vi "MeasureLeq.vi"(0 "channel info left(necessary)":T4={"sensor sensitivity"=12.21, "engineering units"=2, "dB reference"=2e-05, "pregain"=0.0} {"pregain" format="%.2f"; "dB reference" format="%^.1e"; "engineering units" items=["custom..."=0, "V"=1, "A"=21, "C"=30, "pC"=31, "s"=32, "-"=29, "Pa"=2, "N"=20, "g"=3, "m/s^2"=4, "m/s"=5, "m"=6, "mm/s"=12, "mm"=13, "micron/s"=14, "micron"=15, "in/s^2"=7, "in/s"=8, "in"=9, "mil/s"=10, "mil"=11, "rad/s^2"=16, "rad/s"=17, "rad"=18, "deg/s^2"=26, "deg/s"=27, "deg"=28, "RPM"=22, "cycle/s^2"=23, "Hz"=24, "cycle"=25, "strain"=19]; "sensor sensitivity" format="%#_5f"}, 1 "channel info right (necessary)":T4={"sensor sensitivity"=13.0, "engineering units"=2, "dB reference"=2e-05, "pregain"=0.0} caption="channel info right(necessary)" {"pregain" format="%.2f"; "dB reference" format="%^.1e"; "engineering units" items=["custom..."=0, "V"=1, "A"=21, "C"=30, "pC"=31, "s"=32, "-"=29, "Pa"=2, "N"=20, "g"=3, "m/s^2"=4, "m/s"=5, "m"=6, "mm/s"=12, "mm"=13, "micron/s"=14, "micron"=15, "in/s^2"=7, "in/s"=8, "in"=9, "mil/s"=10, "mil"=11, "rad/s^2"=16, "rad/s"=17, "rad"=18, "deg/s^2"=26, "deg/s"=27, "deg"=28, "RPM"=22, "cycle/s^2"=23, "Hz"=24, "cycle"=25, "strain"=19]; "sensor sensitivity" format="%#_5f"}, 3 "sample mode":T9 items=["Finite Samples", "Continuous Samples"], 8 "path":path=path "C:/Users/eeeds/OneDrive/Desktop/white noise30s.wav", 9 "device ID":u32, 10 "task":refnum<k21>, 12 "Amplification":dbl=1.0, 14 "weighting 2":u16(ring)=1 items=["Linear", "A-weighting", "B-weighting", "C-weighting"], 16 "weighting 3":u16(ring)=1 items=["Linear", "A-weighting", "B-weighting", "C-weighting"]) -> (20 "Leq sound level [dB EU] 4":dbl format="%.1f", 22 "max value":dbl, 24 "iterations":i32 caption="Numeric")   [LabVIEW 2019]
uses:
  <vilib>/addons/_NISVFA/_Shared subVIs/Controls/svc_Engineering Units Text Ring.ctl
  <vilib>/addons/_NISVFA/_Shared subVIs/Controls/svc_Window.ctl
  <vilib>/sound2/lvsound2.llb/Sampling Mode.ctl
  <vilib>/addons/_NISVFA/_Shared subVIs/Controls/svc_Weighting Filter Text Ring.ctl
  <vilib>/Utility/error.llb/DialogType.ctl
  <vilib>/DAQmx/read.llb/DAQmx Read (Analog 1D Wfm NChan NSamp).vi
  <vilib>/addons/Sound and Vibration/svt_Calibration/SVL Scale Voltage to EU (N Ch - N Info).vi
  <vilib>/addons/Sound and Vibration/svt_Calibration/SVL Scale Voltage to EU (1 Ch).vi
  <vilib>/addons/_NISVFA/_Shared subVIs/Common/svc_Set SV Channel Info.vi
  <vilib>/addons/_NISVFA/_Shared subVIs/Common/svc_Set SV Channel Info (variant).vi
  <vilib>/addons/_NISVFA/_Shared subVIs/Common/SVL Set dB Reference (variant).vi
  <vilib>/sound2/lvsound2.llb/Sound File Info (path).vi
  GlobalVariable.vi
  <vilib>/DAQmx/miscellaneous.llb/DAQmx Fill In Error Info.vi
  <vilib>/addons/_NISVFA/_Shared subVIs/Common/svc_Engineering Units to Unit Label.vi
  <vilib>/addons/_NISVFA/_Shared subVIs/Common/svc_Compute Scale Factor to Convert V to EU.vi
  <vilib>/addons/_NISVFA/_Shared subVIs/Common/svc_Compute Scale Factor to Convert C to EU.vi
  <vilib>/addons/_NISVFA/_Shared subVIs/Common/svc_Set dB ref if Pascal.vi
  <vilib>/addons/_NISVFA/_Shared subVIs/Common/svc_Caller VI Returned in Error Source.vi
  <vilib>/Waveform/WDTOps.llb/WDT Index Channel DBL.vi
  <vilib>/addons/Sound and Vibration/svt_Weighting/SVT Weighting Filter (1 Ch).vi
  <vilib>/addons/Sound and Vibration/svt_Octave_2014 standard/SVT Third-octave Analysis (1 Ch).vi
  <vilib>/addons/Sound and Vibration/svt_Level/SVL RMS Level (N Ch).vi
  <vilib>/addons/Sound and Vibration/svt_Octave/SVT Third-octave Analysis (N Ch).vi
  <vilib>/addons/_NISVFA/_Baseband FFT/SVFA Power Spectrum (N Ch).vi
  <vilib>/addons/_NISVFA/_Zoom FFT/SVFA Zoom Power Spectrum (N Ch).vi
  <vilib>/addons/_NISVFA/_Subset FFT/SVFA Power Spectrum Subset (N Ch).vi
  <vilib>/addons/_NISVFA/_Baseband FFT/SVFA FFT Spectrum (Mag-Phase) (N Ch).vi
  <vilib>/addons/_NISVFA/_Zoom FFT/SVFA Zoom FFT Spectrum (Mag-Phase) (N Ch).vi
  <vilib>/addons/_NISVFA/_Subset FFT/SVFA FFT Spectrum Subset (Mag-Phase) (N Ch).vi
  <vilib>/addons/_NISVFA/_Baseband FFT/SVFA Power Spectral Density (N Ch).vi
  <vilib>/addons/_NISVFA/_Zoom FFT/SVFA Zoom Power Spectral Density (N Ch).vi
  <vilib>/addons/_NISVFA/_Subset FFT/SVFA Power Spectral Density Subset (N Ch).vi
  <vilib>/addons/Sound and Vibration/svt_Level/SVT Sound Level (1 Ch).vi
  <vilib>/sound2/lvsound2.llb/Sound Output Write (DBL).vi
  <vilib>/addons/Sound and Vibration/svt_Calibration/SoundVib_Calibration.lvlib
  <vilib>/addons/Sound and Vibration/svt_Octave/SoundVib_Octave.lvlib
  <vilib>/addons/Sound and Vibration/svt_Level/SoundVib_VibrationLevel.lvlib
  <vilib>/addons/Sound and Vibration/svt_Weighting/SoundVib_ABCWeighting.lvlib
  <vilib>/addons/Sound and Vibration/svt_Level/SoundVib_SoundLevel.lvlib
  <vilib>/addons/Sound and Vibration/svt_Octave/SoundVib_Octave_2014 standard.lvlib
  <resource>/objmgr/daqmx.rc
panel:
  out "time*10":i16
  in  "channel info right 2(unnecessary)":T2={"weighting filter 2"=0, "custom label"="EU"} {"weighting filter 2" items=["Linear", "A-weighting", "B-weighting", "C-weighting", "ITU-R 468-4", "Dolby", "CCITT", "C-message", "Wb", "Wc", "Wd", "We", "Wf", "Wh", "Wj", "Wk", "Wm", "AES17 20 kHz lowpass", "AES17 40 kHz lowpass", "AES17 20 kHz highpass", "AES17 40 kHz highpass"]}
  in  "channel info left":T5={"sensor sensitivity"=12.21, "engineering units"=2, "dB reference"=2e-05, "custom label"="EU", "weighting filter"=0, "pregain"=0.0} {"pregain" format="%.2f"; "weighting filter" items=["Linear", "A-weighting", "B-weighting", "C-weighting", "ITU-R 468-4", "Dolby", "CCITT", "C-message", "Wb", "Wc", "Wd", "We", "Wf", "Wh", "Wj", "Wk", "Wm", "AES17 20 kHz lowpass", "AES17 40 kHz lowpass", "AES17 20 kHz highpass", "AES17 40 kHz highpass"]; "dB reference" format="%^.1e"; "engineering units" items=["custom..."=0, "V"=1, "A"=21, "C"=30, "pC"=31, "s"=32, "-"=29, "Pa"=2, "N"=20, "g"=3, "m/s^2"=4, "m/s"=5, "m"=6, "mm/s"=12, "mm"=13, "micron/s"=14, "micron"=15, "in/s^2"=7, "in/s"=8, "in"=9, "mil/s"=10, "mil"=11, "rad/s^2"=16, "rad/s"=17, "rad"=18, "deg/s^2"=26, "deg/s"=27, "deg"=28, "RPM"=22, "cycle/s^2"=23, "Hz"=24, "cycle"=25, "strain"=19]; "sensor sensitivity" format="%#_5f"}
  in  "channel info left (unnecessary)":T2={"weighting filter 2"=0, "custom label"="EU"} {"weighting filter 2" items=["Linear", "A-weighting", "B-weighting", "C-weighting", "ITU-R 468-4", "Dolby", "CCITT", "C-message", "Wb", "Wc", "Wd", "We", "Wf", "Wh", "Wj", "Wk", "Wm", "AES17 20 kHz lowpass", "AES17 40 kHz lowpass", "AES17 20 kHz highpass", "AES17 40 kHz highpass"]}
  out "number of channels":dbl
  out "bits per sample":dbl
  out "sample rate":dbl
  in  "channel info right":T5={"sensor sensitivity"=13.0, "engineering units"=2, "dB reference"=2e-05, "custom label"="EU", "weighting filter"=0, "pregain"=0.0} {"pregain" format="%.2f"; "weighting filter" items=["Linear", "A-weighting", "B-weighting", "C-weighting", "ITU-R 468-4", "Dolby", "CCITT", "C-message", "Wb", "Wc", "Wd", "We", "Wf", "Wh", "Wj", "Wk", "Wm", "AES17 20 kHz lowpass", "AES17 40 kHz lowpass", "AES17 20 kHz highpass", "AES17 40 kHz highpass"]; "dB reference" format="%^.1e"; "engineering units" items=["custom..."=0, "V"=1, "A"=21, "C"=30, "pC"=31, "s"=32, "-"=29, "Pa"=2, "N"=20, "g"=3, "m/s^2"=4, "m/s"=5, "m"=6, "mm/s"=12, "mm"=13, "micron/s"=14, "micron"=15, "in/s^2"=7, "in/s"=8, "in"=9, "mil/s"=10, "mil"=11, "rad/s^2"=16, "rad/s"=17, "rad"=18, "deg/s^2"=26, "deg/s"=27, "deg"=28, "RPM"=22, "cycle/s^2"=23, "Hz"=24, "cycle"=25, "strain"=19]; "sensor sensitivity" format="%#_5f"}
  in  "quit 4":bool
  in  "exp avg settings 4":T6={" mode"=enum."Fast", "time constant [ms]"=125.0} {"time constant [ms]" format="%.2f"}
  in  "frequency range 4":T7={"low band"=enum."20 Hz", "high band"=enum."16000 Hz"}
  out "filter settled 3":bool
  out "octave graph 3":T8(graph)
  out "Total Band Power 3":dbl(slide)=nan scale=0.0..100.0
  out "History 3":waveform(dbl)[](graph)
  out "Leq sound level [dB EU] 3":dbl format="%.1f"
  out "unit label 3":string="left dB(A) ref 20.0u Pa" caption="Left"
  out "Exp Avg 3":dbl format="%.1f"
  in  "restart 4":bool
  in  "integration time [s] 2":dbl=10.0 format="%.2f"
  out "Running Leq sound level [dB EU] 4":dbl format="%.1f"
  out "Running Leq sound level [dB EU] 3":dbl format="%.1f"
  in  "integration time [s]":dbl=10.0 format="%.2f"
  out "total number of samples/ch":u32
  in  "scan rate [S/s] 2":dbl=51200.0 min=0.0 format="%.2f"
  out "error 2":bool
  in  "restart 3":bool
  out "Exp Avg 2":dbl format="%.1f"
  out "unit label 2":string="right dB(A) ref 20.0u Pa" caption="Right"
  out "Leq sound level [dB EU] 2":dbl format="%.1f"
  out "History 2":waveform(dbl)[](graph)
  out "Total Band Power 2":dbl(slide)=nan scale=0.0..100.0
  out "octave graph 2":T8(graph)
  out "filter settled 2":bool
  in  "frequency range 3":T7={"low band"=enum."20 Hz", "high band"=enum."16000 Hz"}
  in  "exp avg settings 3":T6={" mode"=enum."Fast", "time constant [ms]"=125.0} {"time constant [ms]" format="%.2f"}
  in  "quit 3":bool
  in  "quit 2":bool
  in  "window":T10=1 items=["None"=0, "Hanning"=1, "Hamming"=2, "Blackman-Harris"=3, "Exact Blackman"=4, "Blackman"=5, "Flat Top"=6, "4 Term B-Harris "=7, "7 Term B-Harris"=8, "Low Sidelobe"=9, "Force"=64, "Exponential"=65, "Blackman Nuttall"=11, "Triangle"=30, "Bartlett-Hanning"=31, "Bohman"=32, "Parzen"=33, "Welch"=34, "Kaiser"=60, "Dolph-Chebyshev"=61, "Gaussian"=62]
  in  "Graph Tab Control":T11(tab)
  out "Power spectrum":cluster{"f0":dbl, "df":dbl, "magnitude":dbl[]}[](graph)
  out "Phase":cluster{"f0":dbl, "df":dbl, "phase":dbl[]}[](graph)
  out "Magnitude":cluster{"f0":dbl, "df":dbl, "magnitude":dbl[]}[](graph)
  out "PSD":cluster{"f0":dbl, "df":dbl, "magnitude":dbl[]}[](graph)
  out "Cursor.Cursor Position:Cursor Y":dbl
  in  "dB On":bool=TRUE
  in  "FFT Type":enum32{"Baseband", "Zoom", "Subset"}(tab)
  out "frequency resolution [Hz]":dbl=50.0 format="%.2f"
  out "time record [ms]":dbl=20.0 format="%.2f"
  in  "zoom settings":T12={"frequency range"={"start frequency"=500.0, "stop frequency"=2000.0}, "window"=enum."Hanning", "number of lines"=400, "% overlap"=0.0} {"% overlap" min=0.0 max=99.0 step=10.0 format="%.2f"; "number of lines" min=1 step=1; "frequency range"."stop frequency" min=0.0 format="%.2f"; "frequency range"."start frequency" min=0.0 format="%.2f"}
  out "zoom FFT":dbl=2.500000055879356 format="%.2f"
  out "baseband FFT":dbl=50.0 format="%.2f"
  out "frequency resolution [Hz] Subset":dbl format="%.2f"
  out "time record [ms] Subset":dbl format="%.2f"
  in  "frequency range 2":T13={"start frequency"=200.0, "stop frequency"=2000.0} {"stop frequency" min=0.0 format="%.2f"; "start frequency" min=0.0 format="%.2f"}
  in  "number of samples":i32=5120 min=128
  out "averages completed":dbl
  out "done":bool
  in  "averaging mode":T14(ring)=enum."RMS averaging"
  in  "number of averages":u32=10
  in  "linear mode":enum16{"One shot", "Auto restart"}(ring)=enum."Auto restart"
  in  "weighting mode":enum16{"Linear", "Exponential"}(ring)
  in  "restart 2":bool
  out "total band powers":dbl[](array[numeric]) format="%.2f"
  in  "exp avg settings 2":T6={" mode"=enum."Fast", "time constant [ms]"=125.0} {"time constant [ms]" format="%.2f"}
  in  "averaging type":T15(ring)
  out "RMS levels [EU rms]":dbl[](array[numeric]) format="%.2f"
  # "For HATS4128C:\nLeft sensor sensitivity: 12.60, Pregain: 2.60 dB\nRight sensor sensitivity: 12.60, Pregain: 3.00 dB\n\nFor GRAS 45BB:\nLeft sensor sensitivity: 12.21, Pregain: 3.30 dB\nRight sensor sensitivity: 13.00, Pregain: 1.30 dB\n\nAlso, remember to change the following:\n1) Number of samples/ch\n2) Path of file for calibration\n3) Press CTRL+E to open the loop and change the loop iterations number to 10 x length of file to be calibrated/s\n4) Change \"physical channels 2\" to the name of the NiDAQ being used (Reselect active module)\n\nTo run calibration:\n1) Press the \"Run\" button (white arrow at top toolbar)\n2) Change the settings to: Terminal config = Pseudodifferential, Coupling = AC, Sensor Excitation = Disable (uncheck box)\n\nTo record using GRAS microphone:\n1) Press the \"Run\" button (white arrow at top toolbar)\n2) Change the settings to: Terminal config = Pseudodifferential, Coupling = AC, Sensor Excitation = Enable (check box), Excitation value = 2m\n\nWhen using Sound Blaster Creative E5 for playback, please make sure that the volume is set to 40 and that it is indeed the playback device (on Windows)."
  # "Please change this to length of\ntrack/s x sampling frequency/Hz"
  # "Average Leq \n(Both Channels)"
  # "Note that if the amplification value here is x, then the SPL level of the playback has been increased by 20ln(x) dB. Use Audacity to modify the peak SPL level of the file to calibrate it, using this amplification level."
  # "Change this to the file you want to calibrate.\nRight click and select \"Data Operatons\" ->\n\"Make Current Value Defualt\" to save the file\nname here"
  # "Increase number of samples to improve frequency resolution (for a given sampling frequency)"
  # "frequency resolution [Hz]"
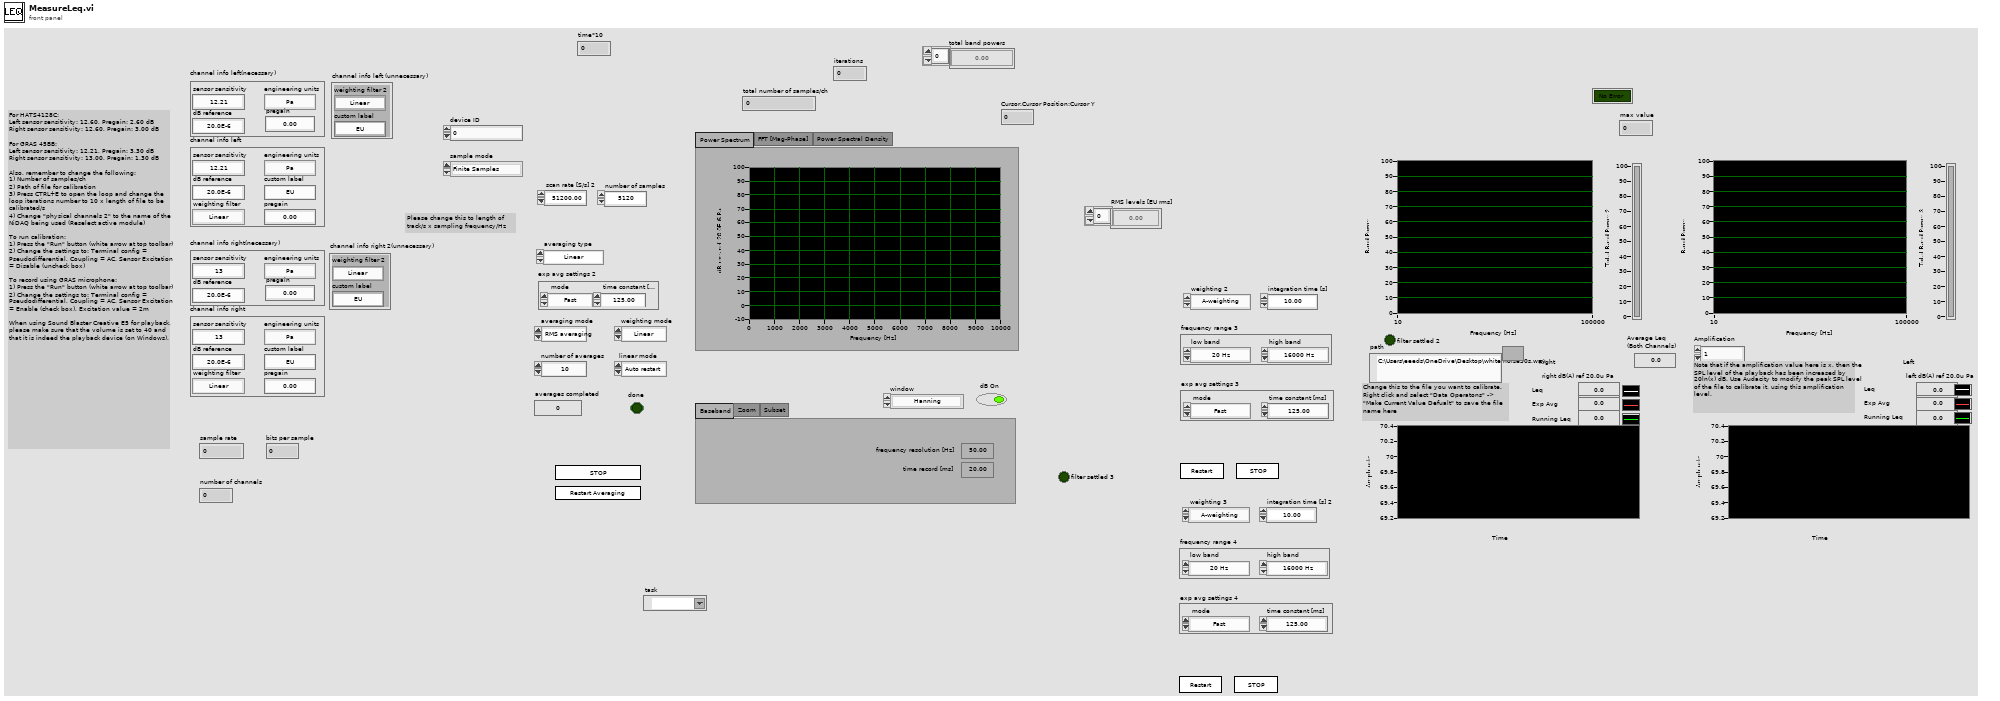
[diagram p1: front panel]
types:
  T1 = typedef "svc_Weighting Filter Text Ring.ctl" = u16
  T2 = cluster{"weighting filter 2":T1, "custom label":string}
  T3 = typedef "svc_Engineering Units Text Ring.ctl" = u16
  T4 = cluster{"sensor sensitivity":dbl, "engineering units":T3, "dB reference":dbl, "pregain":dbl}
  T5 = cluster{"sensor sensitivity":dbl, "engineering units":T3, "dB reference":dbl, "custom label":string, "weighting filter":T1, "pregain":dbl}
  T6 = cluster{" mode":enum16{"Slow", "Fast", "Impulse", "Custom"}, "time constant [ms]":dbl}
  T7 = cluster{"low band":enum16{"20 Hz", "25 Hz", "31.5 Hz", "40 Hz", "50 Hz", "63 Hz", "80 Hz", "100 Hz", "125 Hz", "160 Hz", "200 Hz", "250 Hz", "315 Hz", "400 Hz", "500 Hz", "630 Hz", "800 Hz", "1000 Hz", "1250 Hz", "1600 Hz", "2000 Hz", "2500 Hz", "3150 Hz", "4000 Hz", "5000 Hz", "6300 Hz", "8000 Hz", "10000 Hz", "12500 Hz", "16000 Hz", "20000 Hz"}, "high band":enum16{"20 Hz", "25 Hz", "31.5 Hz", "40 Hz", "50 Hz", "63 Hz", "80 Hz", "100 Hz", "125 Hz", "160 Hz", "200 Hz", "250 Hz", "315 Hz", "400 Hz", "500 Hz", "630 Hz", "800 Hz", "1000 Hz", "1250 Hz", "1600 Hz", "2000 Hz", "2500 Hz", "3150 Hz", "4000 Hz", "5000 Hz", "6300 Hz", "8000 Hz", "10000 Hz", "12500 Hz", "16000 Hz", "20000 Hz"}}
  T8 = cluster{"nominal frequencies [Hz]":dbl[], "band power":dbl[]}
  T9 = typedef "Sampling Mode.ctl" = i32
  T10 = typedef "svc_Window.ctl" = u32
  T11 = enum32{"Power Spectrum", "FFT [Mag-Phase]", "Power Spectral Density"}
  T12 = cluster{"frequency range":cluster{"start frequency":dbl, "stop frequency":dbl}, "window":enum16{"None ", "Hanning", "Hamming", "Blackman-Harris", "Exact Blackman", "Blackman", "Flat Top", "4 Term B-Harris ", "7 Term B-Harris", "Low Sidelobe"}, "number of lines":i32, "% overlap":dbl}
  T13 = cluster{"start frequency":dbl, "stop frequency":dbl}
  T14 = enum16{"No averaging", "Vector averaging", "RMS averaging", "Peak hold"}
  T15 = enum16{"Linear", "Exponential", "Equal confidence", "Peak"}
  T16 = cluster{"Leq":bool, "Running Leq":bool, "Exponential":bool, "Peak":bool}
  T17 = cluster{"averaging mode":enum16{"No averaging", "Vector averaging", "RMS averaging", "Peak hold"}, "weighting mode":enum16{"Linear", "Exponential"}, "number of averages":u32, "linear mode":enum16{"One shot", "Auto restart"}}
  T18 = cluster{"dB On (T)":bool, "unwrap phase (F)":bool, "convert to degree (T)":bool}
  T19 = typedef "Sound Data Format.ctl" = cluster{"sample rate (S/s)":dbl, "number of channels":i32, "bits per sample":i32}
  T20 = typedef "DialogType.ctl" = u16
  T21 = typedef "Sound Output Task ID.ctl" = u32
  T22 = cluster{"sensor sensitivity":dbl, "engineering units":T3, "dB reference":dbl, "custom label":string, "weighting filter":T1, "pregain":dbl}[]
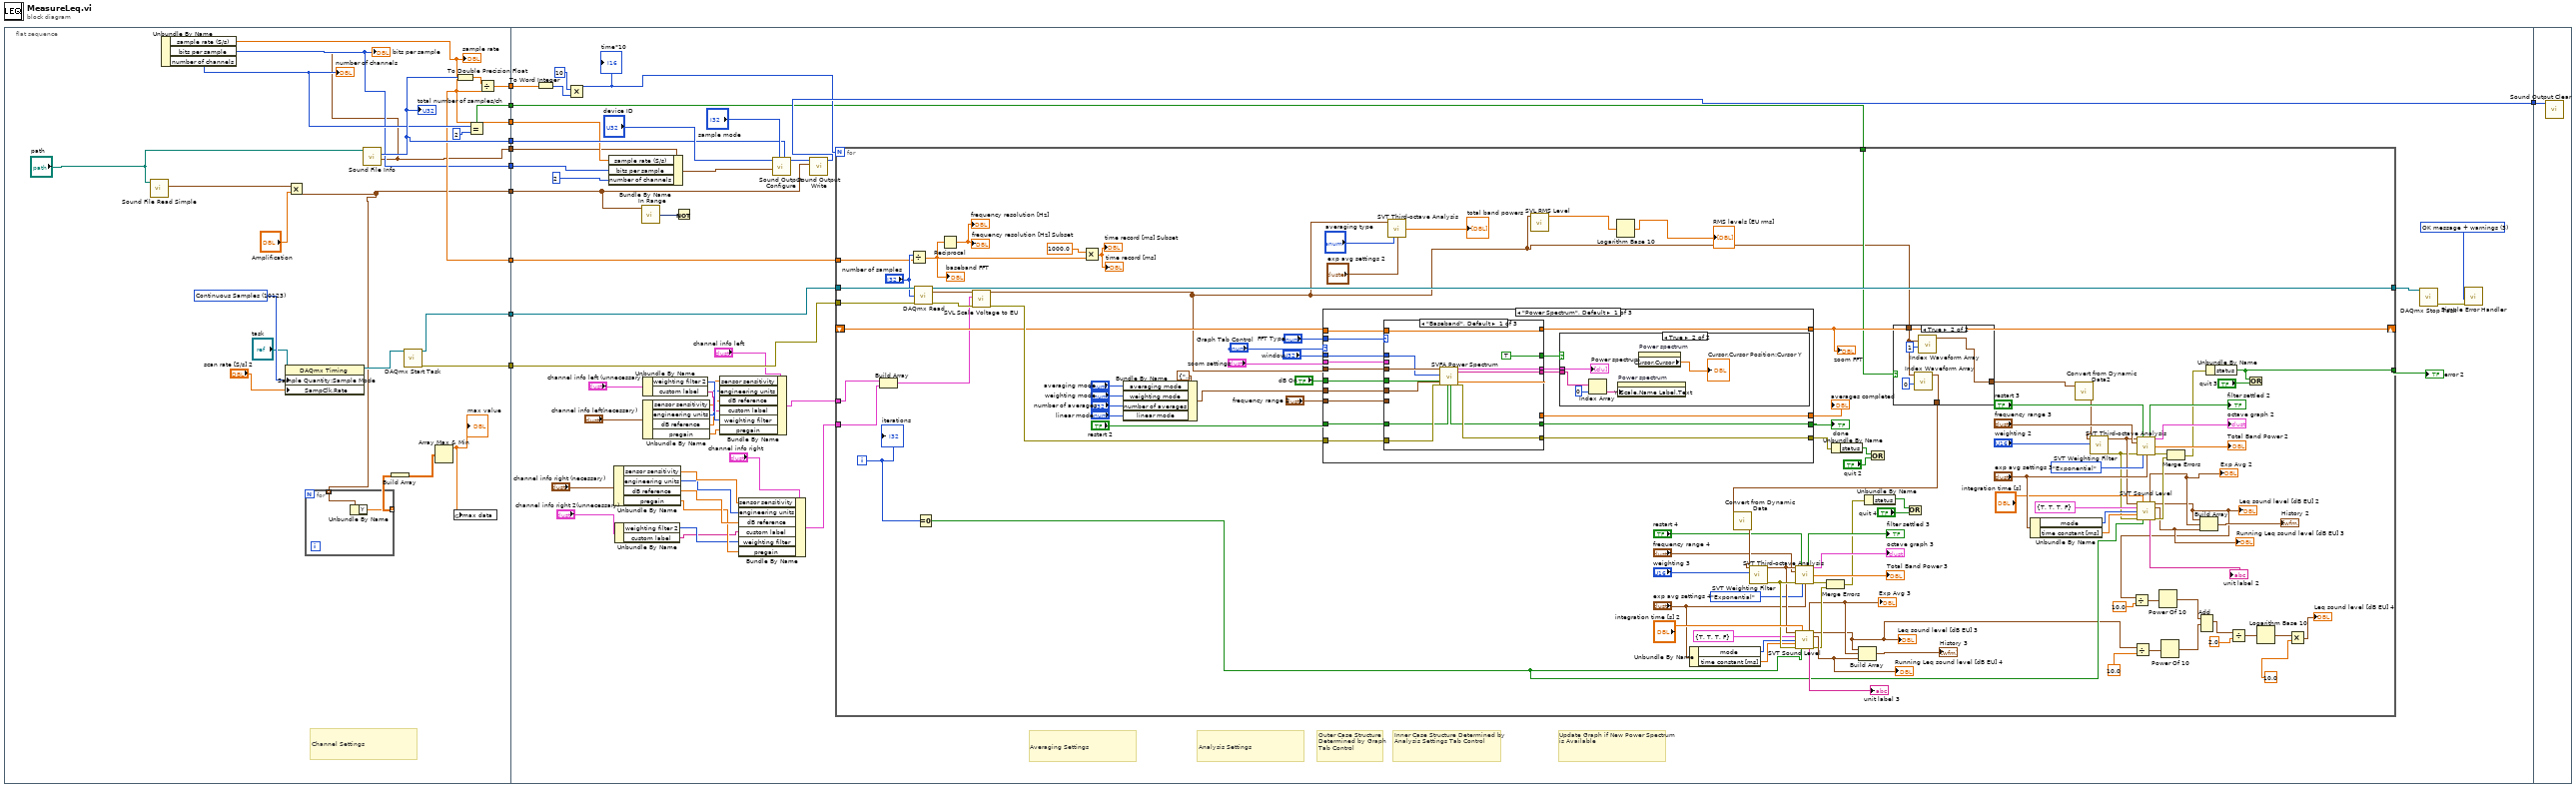
[diagram p0: block diagram]
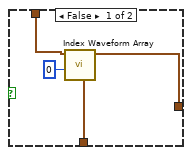
[diagram p2: hidden frame]
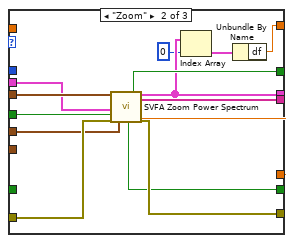
[diagram p4: hidden frame]
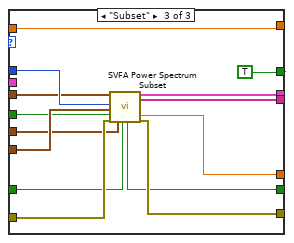
[diagram p5: hidden frame]
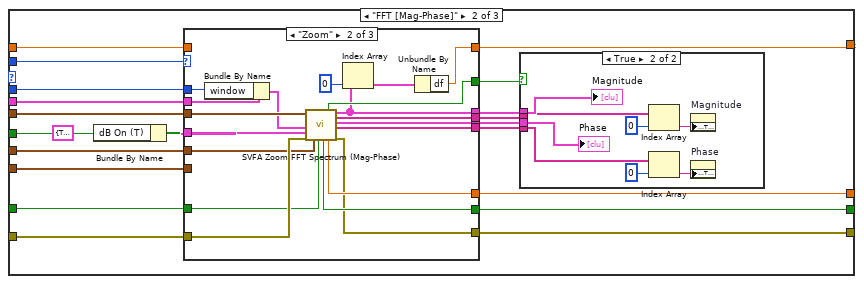
[diagram p6: hidden frame]
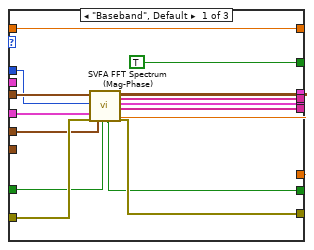
[diagram p8: hidden frame]
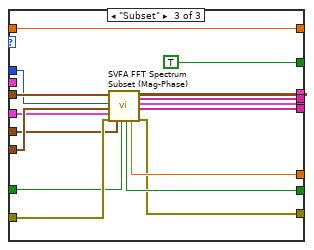
[diagram p9: hidden frame]
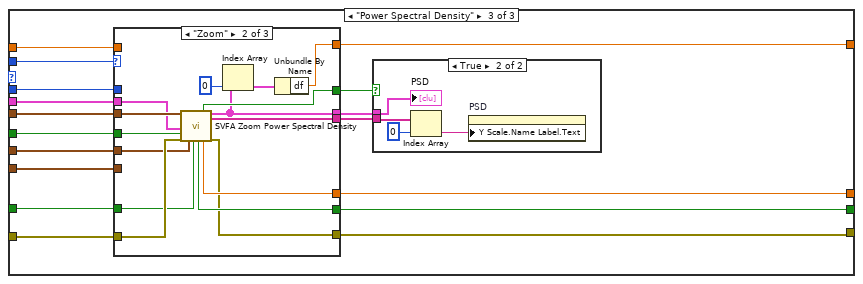
[diagram p10: hidden frame]
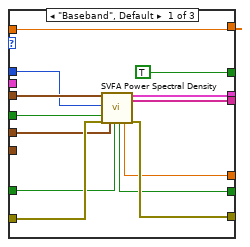
[diagram p12: hidden frame]
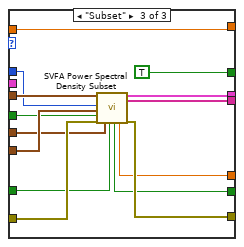
[diagram p13: hidden frame]
diagram:
  n1 = flat-sequence {
    tunnel: [w16] -> w11
    tunnel: [w33] -> w10
    tunnel: [w32] -> w9
    tunnel: [w29] -> w7
    tunnel: [w28] -> w6
    tunnel: [w19] -> w5
    tunnel: [w21] -> w4
    tunnel: [w19] -> w3
    tunnel: [w18] -> w2
    tunnel: [w17] -> w1
    tunnel: w11 -> [w41]
    tunnel: w10 -> [w73]
    tunnel: w9 -> [w72]
    tunnel: [w70] -> w8
    tunnel: w7 -> [w48]
    tunnel: w6 -> [w44]
    tunnel: w5 -> [w43]
    tunnel: w4 -> [w42]
    tunnel: w3 -> [w40]
    tunnel: w2 -> [w39]
    tunnel: w1 -> [w37]
    tunnel: w8 -> [w402]
    frame #0 {
      w15 = 10123 items=["Finite Samples"=10178, "Continuous Samples"=10123] ("sample mode")
      # "Channel Settings"
      n2 = call <vilib>:"Sound File Read Simple.vi"("path"="path") -> ("data"=w20:waveform(dbl)[])  [unwired: 7 in, 3 out]
      n3 = property class="DAQmx Timing"(reference="task", "Sample Quantity:Sample Mode"=w15, "SampClk.Rate"="scan rate [S/s] 2") -> (reference out=w24:refnum<k21>)  [unwired: 1 in, 1 out]
      n4 = Multiply(x=w20, y="Amplification") -> (x*y=w16:waveform(dbl)[])
      n5 = for {
        tunnel: [w35] -> w27 mode=indexing
        tunnel: w16 -> [w34] mode=indexing
        n6 = Unbundle By Name(w34) -> ("Y"=w35:dbl[])
      }
      n7 = call-poly <vilib>:"Sound File Info.vi"("path"="path") -> ("sound format"=w17:T19, "total number of samples/ch"=w28:u32)  [unwired: 7 in, 2 out]
      "total number of samples/ch" <- w28
      n8 = Unbundle By Name(w17) -> ("sample rate (S/s)"=w19:dbl, "bits per sample"=w18:i32, "number of channels"=w23:i32)
      "sample rate" <- w19
      "bits per sample" <- w18
      "number of channels" <- w23
      n9 = Build Array(w27) -> (w26:dbl[][][])
      n10 = call <vilib>:"DAQmx Start Task.vi"("task/channels in"=w24) -> ("task out"=w33:refnum<k21>, "error out"=w32:errorcluster)  [unwired: 13 in]
      n11 = Array Max & Min(array=w26) -> (max value=w25:dbl)  [unwired: 3 out]
      "max value" <- w25
      n12 = global write "GlobalVariable.vi" "max data"(w25) -> ()
      n13 = To Double Precision Float(number=w28) -> (double precision float=w30:dbl)
      n14 = Equal?(x=w23, y=2) -> (x = y?=w21:bool)
      n15 = Divide(x=w30, y=w19) -> (x/y=w29:dbl)
    }
    frame #1 {
      w79 = T20 3 items=["no dialog", "OK message", "continue or stop message", "OK message + warnings", "continue/stop + warnings"] ("type of dialog (OK msg:1)")
      # "Update Graph if New Power Spectrum is Available"
      # "Inner Case Structure Determined by Analysis Settings Tab Control"
      # "Analysis Settings"
      # "Outer Case Structure Determined by Graph Tab Control"
      # "Averaging Settings"
      n16 = To Word Integer(number=w48) -> (16bit integer=w47:i16)
      n17 = Multiply(x=i16 10, y=w47) -> (x*y=w46:i16)
      "time*10" <- w46
      n18 = Bundle By Name(cluster=w37, "sample rate (S/s)"=w40, "bits per sample"=w39, "number of channels"=2) -> (w36:T19)
      n19 = Unbundle By Name("channel info right (necessary)") -> ("sensor sensitivity"=w58:dbl, "engineering units"=w57:T3, "dB reference"=w56:dbl, "pregain"=w55:dbl)
      n20 = Unbundle By Name("channel info right 2(unnecessary)") -> ("weighting filter 2"=w54:T1, "custom label"=w53:string)
      n21 = call "In Range"("Operand 1"=w41) -> ("Result"=w69:dynamicdata)  [unwired: 9 in, 1 out]
      n22 = Unbundle By Name("channel info left (unnecessary)") -> ("weighting filter 2"=w64:T1, "custom label"=w63:string)
      n23 = Unbundle By Name("channel info left(necessary)") -> ("sensor sensitivity"=w62:dbl, "engineering units"=w61:T3, "dB reference"=w60:dbl, "pregain"=w59:dbl)
      n24 = Not(x=w69) -> ()  [unwired: 1 out]
      n25 = Bundle By Name(cluster="channel info left", "sensor sensitivity"=w62, "engineering units"=w61, "dB reference"=w60, "custom label"=w63, "weighting filter"=w64, "pregain"=w59) -> (w49:T5)
      n26 = Bundle By Name(cluster="channel info right", "sensor sensitivity"=w58, "engineering units"=w57, "dB reference"=w56, "custom label"=w53, "weighting filter"=w54, "pregain"=w55) -> (w50:T5)
      n27 = call <vilib>:"Sound Output Configure.vi"("number of samples/ch"=w44, "sample mode"="sample mode", "sound format"=w36, "device ID"="device ID") -> ("task ID"=w74:T21)  [unwired: 6 in, 1 out]
      n28 = call-poly <vilib>:"Sound Output Write.vi"("data"=w41, "task ID"=w74) -> ("task ID out"=w70:T21)  [unwired: 8 in, 1 out]
      n29 = for {
        N: w46 -> [_]
        shift-right: [w178] -> _
        shift-left: _ -> [w181]
        tunnel: [w129] -> w77
        tunnel: w73 -> [w173]
        tunnel: w72 -> [w170]
        tunnel: [w133] -> w76
        tunnel: w49 -> [w102]
        tunnel: w50 -> [w103]
        tunnel: w43 -> [w97]
        tunnel: w42 -> [w96]
        i -> [w99]
        w130 = T20 3 items=["no dialog", "OK message", "continue or stop message", "OK message + warnings", "continue/stop + warnings"] ("type of dialog (OK msg:1)")
        n30 = Build Array(w102, w103) -> (w101:T22)
        n31 = Divide(x="number of samples", y=w97) -> (x/y=w179:dbl)
        "baseband FFT" <- w179
        n32 = call-poly <vilib>:"DAQmx Read.vi"("task/channels in"=w173, "number of samples per channel"="number of samples", "error in"=w170) -> ("task out"=w129:refnum<k21>, "data"=w174:waveform(dbl)[], "error out"=w171:errorcluster)  [unwired: 10 in]
        n33 = Equal To 0?(x=w99) -> (x = 0?=w98:bool)
        n34 = Reciprocal(x=w179) -> (1/x=→"frequency resolution [Hz]" →"frequency resolution [Hz] Subset":dbl)
        n35 = call-poly <vilib>:"SVL Scale Voltage to EU.vi"("error in (no error)"=w171, "channel info"=w101, "signals [V]"=w174) -> ("error out"=w187:errorcluster, "scaled signals [EU]"=w95:waveform(dbl)[])  [unwired: 6 in, 1 out]
        n36 = Multiply(x=1000.0 ("y"), y=w179) -> (x*y=→"time record [ms]" →"time record [ms] Subset":dbl)
        n37 = Bundle By Name(cluster=T17 {"averaging mode"=enum."RMS averaging", "weighting mode"=enum."Exponential", "number of averages"=10, "linear mode"=enum."Auto restart"} ("averaging parameters"), "averaging mode"="averaging mode", "weighting mode"="weighting mode", "number of averages"="number of averages", "linear mode"="linear mode") -> (w164:T17)
        n38 = case shown="\"Power Spectrum\", Default" "Graph Tab Control" {
          tunnel: w187 -> [w212 w280 w354]
          tunnel: w95 -> [w213 w279 w355]
          tunnel: [w211 w278 w353] -> w160
          tunnel: "window" -> [w210 w262 w352]
          tunnel: w164 -> [w209 w277 w351]
          tunnel: "restart 2" -> [w208 w276 w339]
          tunnel: [w206 w275 w350] -> w162
          tunnel: [w205 w274 w349] -> w163
          tunnel: "dB On" -> [w204 w272 w343]
          tunnel: "FFT Type" -> [w202 w267 w345]
          tunnel: [w201 w264 w342] -> w178
          tunnel: w181 -> [w199 w263 w341]
          tunnel: "zoom settings" -> [w198 w266 w344]
          tunnel: "frequency range 2" -> [w197 w261 w340]
          frame "Power Spectrum", Default {
            n39 = case shown="\"Baseband\", Default" w202 {
              tunnel: w213 -> [w231 w245 w257]
              tunnel: w212 -> [w230 w244 w256]
              tunnel: [w229 w243 w254] -> w211
              tunnel: w210 -> [w228 _ w258]
              tunnel: w209 -> [w227 w232 w246]
              tunnel: w208 -> [w226 _ w248]
              tunnel: [w225 w234 w255] -> w207
              tunnel: [w224 w238 w249] -> w206
              tunnel: [w223 w237 w250] -> w205
              tunnel: w204 -> [w222 w236 w247]
              tunnel: [w221 w240 w253] -> w203
              tunnel: [w219 w242 w251] -> w201
              tunnel: [TRUE ("new spectrum available") w241 TRUE ("new spectrum available")] -> w200
              tunnel: w199 -> [w219 _ w251]
              tunnel: w198 -> [_ w239 _]
              tunnel: w197 -> [_ _ w259]
              frame "Baseband", Default {
                n40 = call-poly <vilib>:"SVFA Power Spectrum.vi"("scaled signals [EU]"=w231, "window"=w228, "dB On (T)"=w222, "error in (no error)"=w230, "averaging parameters"=w227, "restart averaging (F)"=w226) -> ("averaging done"=w224:bool, "averages completed"=w223:dbl, "power spectra [dB EU]"=w225:cluster{"f0":dbl, "df":dbl, "magnitude":dbl[]}[], "unit labels"=w221:string[], "error out"=w229:errorcluster)  [unwired: 8 in, 1 out]
              }
              frame "Zoom" {
                n41 = call-poly <vilib>:"SVFA Zoom Power Spectrum.vi"("scaled signals [EU]"=w245, "zoom settings"=w239, "dB On (T)"=w236, "error in (no error)"=w244, "averaging parameters"=w232) -> ("averaging done"=w238:bool, "new spectrum available"=w241:bool, "averages completed"=w237:dbl, "power spectra [dB EU]"=w234:cluster{"f0":dbl, "df":dbl, "magnitude":dbl[]}[], "unit labels"=w240:string[], "error out"=w243:errorcluster)  [unwired: 8 in, 1 out]
                n42 = Index Array(array=w234, index=0) -> (element=w235:cluster{"f0":dbl, "df":dbl, "magnitude":dbl[]})
                n43 = Unbundle By Name(w235) -> ("df"=w242:dbl)
              }
              frame "Subset" {
                n44 = call-poly <vilib>:"SVFA Power Spectrum Subset.vi"("scaled signals [EU]"=w257, "window"=w258, "frequency range"=w259, "dB On (T)"=w247, "error in (no error)"=w256, "averaging parameters"=w246, "restart averaging (F)"=w248) -> ("averaging done"=w249:bool, "averages completed"=w250:dbl, "power spectra [dB EU]"=w255:cluster{"f0":dbl, "df":dbl, "magnitude":dbl[]}[], "unit labels"=w253:string[], "error out"=w254:errorcluster)  [unwired: 7 in, 1 out]
              }
            }
            n45 = case shown="True" w200 {
              tunnel: w207 -> [_ w218]
              tunnel: w203 -> [_ w217]
              frame False {
              }
              frame True {
                n46 = Index Array(array=w217, index=0) -> (element=w215:string)
                n47 = property on="Power spectrum" class="WFGraph (strict)"("Y Scale.Name Label.Text"=w215) -> ()  [unwired: 2 in, 2 out]
                n48 = property on="Power spectrum" class="WFGraph (strict)"() -> ("Cursor.Cursor Y"=→"Cursor.Cursor Position:Cursor Y":dbl)  [unwired: 2 in, 2 out]
                "Power spectrum" <- w218
              }
            }
          }
          frame "FFT [Mag-Phase]" {
            n49 = Bundle By Name(cluster=T18 {"dB On (T)"=TRUE, "unwrap phase (F)"=FALSE, "convert to degree (T)"=TRUE} ("view"), "dB On (T)"=w272) -> (w271:T18)
            n50 = case shown="\"Zoom\"" w267 {
              tunnel: w280 -> [w303 w319 w337]
              tunnel: w279 -> [w302 w322 w338]
              tunnel: [w301 w315 w332] -> w278
              tunnel: w277 -> [w300 w318 w324]
              tunnel: w276 -> [w299 w309 w335]
              tunnel: [w298 w317 w334] -> w275
              tunnel: [w297 w316 w333] -> w274
              tunnel: w262 -> [w296 w307 w323]
              tunnel: [w295 w306 w331] -> w273
              tunnel: w271 -> [w294 w320 w327]
              tunnel: [w293 w313 w325] -> w260
              tunnel: [w292 w314 w328] -> w270
              tunnel: [w291 w312 w330] -> w268
              tunnel: w266 -> [_ w321 _]
              tunnel: [TRUE ("new spectrum available") w311 TRUE ("new spectrum available")] -> w265
              tunnel: [w289 w310 w326] -> w264
              tunnel: w263 -> [w289 _ w326]
              tunnel: w261 -> [_ _ w336]
              frame "Baseband", Default {
                n51 = call-poly <vilib>:"SVFA FFT Spectrum (Mag-Phase).vi"("scaled signals [EU]"=w302, "window"=w296, "view"=w294, "error in (no error)"=w303, "averaging parameters"=w300, "restart averaging (F)"=w299) -> ("averaging done"=w298:bool, "averages completed"=w297:dbl, "magnitudes [dB EU]"=w295:cluster{"f0":dbl, "df":dbl, "magnitude":dbl[]}[], "magnitude unit labels"=w292:string[], "phases [degrees]"=w293:cluster{"f0":dbl, "df":dbl, "phase":dbl[]}[], "phase unit labels"=w291:string[], "error out"=w301:errorcluster)  [unwired: 6 in, 1 out]
              }
              frame "Zoom" {
                n52 = Bundle By Name(cluster=w321, "window"=w307) -> (w308:T12)
                n53 = call-poly <vilib>:"SVFA Zoom FFT Spectrum (Mag-Phase).vi"("scaled signals [EU]"=w322, "zoom settings"=w308, "view"=w320, "error in (no error)"=w319, "averaging parameters"=w318, "restart averaging (F)"=w309) -> ("averaging done"=w317:bool, "new spectrum available"=w311:bool, "averages completed"=w316:dbl, "magnitudes [dB EU]"=w306:cluster{"f0":dbl, "df":dbl, "magnitude":dbl[]}[], "magnitude unit labels"=w314:string[], "phases [degrees]"=w313:cluster{"f0":dbl, "df":dbl, "phase":dbl[]}[], "phase unit labels"=w312:string[], "error out"=w315:errorcluster)  [unwired: 5 in, 1 out]
                n54 = Index Array(array=w306, index=0) -> (element=w305:cluster{"f0":dbl, "df":dbl, "magnitude":dbl[]})
                n55 = Unbundle By Name(w305) -> ("df"=w310:dbl)
              }
              frame "Subset" {
                n56 = call-poly <vilib>:"SVFA FFT Spectrum Subset (Mag-Phase).vi"("scaled signals [EU]"=w338, "window"=w323, "frequency range"=w336, "view"=w327, "error in (no error)"=w337, "averaging parameters"=w324, "restart averaging (F)"=w335) -> ("averaging done"=w334:bool, "averages completed"=w333:dbl, "magnitudes [dB EU]"=w331:cluster{"f0":dbl, "df":dbl, "magnitude":dbl[]}[], "magnitude unit labels"=w328:string[], "phases [degrees]"=w325:cluster{"f0":dbl, "df":dbl, "phase":dbl[]}[], "phase unit labels"=w330:string[], "error out"=w332:errorcluster)  [unwired: 5 in, 1 out]
              }
            }
            n57 = case shown="True" w265 {
              tunnel: w273 -> [_ w288]
              tunnel: w270 -> [_ w283]
              tunnel: w268 -> [_ w286]
              tunnel: w260 -> [_ w287]
              frame False {
              }
              frame True {
                n58 = Index Array(array=w283, index=0) -> (element=w281:string)
                n59 = Index Array(array=w286, index=0) -> (element=w284:string)
                n60 = property on="Magnitude" class="WFGraph (strict)"("Y Scale.Name Label.Text"=w281) -> ()  [unwired: 2 in, 2 out]
                n61 = property on="Phase" class="WFGraph (strict)"("Y Scale.Name Label.Text"=w284) -> ()  [unwired: 2 in, 2 out]
                "Magnitude" <- w288
                "Phase" <- w287
              }
            }
          }
          frame "Power Spectral Density" {
            n62 = case shown="\"Zoom\"" w345 {
              tunnel: w355 -> [w372 w387 w400]
              tunnel: w354 -> [w371 w386 w393]
              tunnel: [w370 w379 w401] -> w353
              tunnel: w352 -> [w369 _ w392]
              tunnel: w351 -> [w368 w383 w389]
              tunnel: w339 -> [w367 w382 w388]
              tunnel: [w366 w381 w394] -> w350
              tunnel: [w365 w380 w395] -> w349
              tunnel: [w364 w375 w398] -> w348
              tunnel: [w363 w378 w397] -> w347
              tunnel: [TRUE ("new spectrum available") w377 TRUE ("new spectrum available")] -> w346
              tunnel: w344 -> [_ w385 _]
              tunnel: w343 -> [w360 w384 w390]
              tunnel: [w362 w376 w399] -> w342
              tunnel: w341 -> [w362 _ w399]
              tunnel: w340 -> [_ _ w391]
              frame "Baseband", Default {
                n63 = call-poly <vilib>:"SVFA Power Spectral Density.vi"("scaled signals [EU]"=w372, "window"=w369, "dB On (F)"=w360, "error in (no error)"=w371, "averaging parameters"=w368, "restart averaging (F)"=w367) -> ("averaging done"=w366:bool, "averages completed"=w365:dbl, "power spectral densities [EU^2 rms / Hz]"=w364:cluster{"f0":dbl, "df":dbl, "magnitude":dbl[]}[], "unit labels"=w363:string[], "error out"=w370:errorcluster)  [unwired: 8 in, 1 out]
              }
              frame "Zoom" {
                n64 = call-poly <vilib>:"SVFA Zoom Power Spectral Density.vi"("scaled signals [EU]"=w387, "zoom settings"=w385, "dB On (T)"=w384, "error in (no error)"=w386, "averaging parameters"=w383, "restart averaging (F)"=w382) -> ("averaging done"=w381:bool, "new spectrum available"=w377:bool, "averages completed"=w380:dbl, "power spectral densities [EU^2 rms / Hz]"=w375:cluster{"f0":dbl, "df":dbl, "magnitude":dbl[]}[], "unit labels"=w378:string[], "error out"=w379:errorcluster)  [unwired: 7 in, 1 out]
                n65 = Index Array(array=w375, index=0) -> (element=w374:cluster{"f0":dbl, "df":dbl, "magnitude":dbl[]})
                n66 = Unbundle By Name(w374) -> ("df"=w376:dbl)
              }
              frame "Subset" {
                n67 = call-poly <vilib>:"SVFA Power Spectral Density Subset.vi"("scaled signals [EU]"=w400, "window"=w392, "frequency range"=w391, "dB On (T)"=w390, "error in (no error)"=w393, "averaging parameters"=w389, "restart averaging (F)"=w388) -> ("averaging done"=w394:bool, "averages completed"=w395:dbl, "power spectral densities [EU^2 rms / Hz]"=w398:cluster{"f0":dbl, "df":dbl, "magnitude":dbl[]}[], "unit labels"=w397:string[], "error out"=w401:errorcluster)  [unwired: 7 in, 1 out]
              }
            }
            n68 = case shown="True" w346 {
              tunnel: w348 -> [_ w359]
              tunnel: w347 -> [_ w358]
              frame False {
              }
              frame True {
                n69 = Index Array(array=w358, index=0) -> (element=w356:string)
                n70 = property on="PSD" class="WFGraph (strict)"("Y Scale.Name Label.Text"=w356) -> ()  [unwired: 2 in, 2 out]
                "PSD" <- w359
              }
            }
          }
        }
        "zoom FFT" <- w178
        "averages completed" <- w163
        "done" <- w162
        n71 = call-poly <vilib>:"SVT Third-octave Analysis.vi"("scaled signals [EU]"=w95, "averaging type"="averaging type", "exp avg settings"="exp avg settings 2") -> ("total band powers"=→"total band powers":dbl[])  [unwired: 7 in, 5 out]
        n72 = call-poly <vilib>:"SVL RMS Level.vi"("scaled signals [EU]"=w95) -> ("RMS levels [EU rms]"=w155:dbl[])  [unwired: 8 in, 2 out]
        n73 = Logarithm Base 10(1:w155) -> (0:→"RMS levels [EU rms]":dbl[])
        n74 = Unbundle By Name("exp avg settings 4") -> ("mode"=w115:enum16{"Slow", "Fast", "Impulse", "Custom"}, "time constant [ms]"=w116:dbl)
        n75 = Unbundle By Name(w160) -> ("status"=w186:bool)
        n76 = Or(x=w186, y="quit 2") -> ()  [unwired: 1 out]
        n77 = case shown="True" w96 {
          tunnel: w95 -> [w191 w196]
          tunnel: [w189 w193] -> w128
          tunnel: [w189 w192] -> w94
          frame False {
            n78 = call-poly <vilib>:"Index Waveform Array.vi"("index"=0, "waveform array"=w191) -> ("waveform"=w189:waveform(dbl))  [unwired: 8 in, 1 out]
          }
          frame True {
            n79 = call-poly <vilib>:"Index Waveform Array.vi"("index"=0, "waveform array"=w196) -> ("waveform"=w192:waveform(dbl))  [unwired: 8 in, 1 out]
            n80 = call-poly <vilib>:"Index Waveform Array.vi"("index"=1, "waveform array"=w196) -> ("waveform"=w193:waveform(dbl))  [unwired: 8 in, 1 out]
          }
        }
        n81 = call "Convert from Dynamic Data"("Dynamic Data Type"=w94) -> ("Waveform"=w124:waveform(dbl))  [unwired: 3 in]
        n82 = call-poly <vilib>:"SVT Weighting Filter.vi"("weighting"="weighting 3", "scaled signal [EU]"=w124) -> ("error out"=w120:errorcluster, "weighted signal [EU]"=w114:waveform(dbl))  [unwired: 7 in]
        n83 = call-poly <vilib>:"SVT Third-octave Analysis.vi"("scaled signal [EU]"=w114, "restart averaging (F)"="restart 4", "frequency range"="frequency range 4", "error in (no error)"=w120, "averaging type"=T15."Exponential", "exp avg settings"="exp avg settings 4") -> ("filter settled"=→"filter settled 3":bool, "octave spectrum"=→"octave graph 3":T8, "total band power"=→"Total Band Power 3":dbl, "error out"=w122:errorcluster)  [unwired: 4 in, 2 out]
        n84 = call-poly <vilib>:"SVT Sound Level.vi"("scaled signal [EU]"=w114, "integration time [s]"="integration time [s] 2", "measurement selection"=T16 {"Leq"=TRUE, "Running Leq"=TRUE, "Exponential"=TRUE, "Peak"=FALSE}, "exponential mode"=w115, "time constant [ms]"=w116, "error in (no error)"=w120, "restart averaging (F)"=w98) -> ("exp avg sound level [dB EU]"=w118:waveform(dbl), "Leq sound level [dB EU]"=w93:waveform(dbl), "running Leq sound level [dB EU]"=w127:waveform(dbl), "unit label"=→"unit label 3":string, "error out"=w121:errorcluster)  [unwired: 3 in, 1 out]
        "Leq sound level [dB EU] 3" <- w93
        "Exp Avg 3" <- w118
        "Running Leq sound level [dB EU] 4" <- w127
        n85 = Merge Errors(w122, w121) -> (w104:errorcluster)
        n86 = Build Array(w93, w118, w127) -> (→"History 3":waveform(dbl)[])
        n87 = Unbundle By Name(w104) -> ("status"=w125:bool)
        n88 = Or(x=w125, y="quit 4") -> ()  [unwired: 1 out]
        n89 = Unbundle By Name("exp avg settings 3") -> ("mode"=w143:enum16{"Slow", "Fast", "Impulse", "Custom"}, "time constant [ms]"=w142:dbl)
        n90 = call "Convert from Dynamic Data2"("Dynamic Data Type"=w128) -> ("Waveform"=w134:waveform(dbl))  [unwired: 3 in]
        n91 = call-poly <vilib>:"SVT Weighting Filter.vi"("weighting"="weighting 2", "scaled signal [EU]"=w134) -> ("error out"=w139:errorcluster, "weighted signal [EU]"=w144:waveform(dbl))  [unwired: 7 in]
        n92 = Divide(x=w93, y=10.0) -> (x/y=w88:waveform(dbl))
        n93 = call-poly <vilib>:"SVT Third-octave Analysis.vi"("scaled signal [EU]"=w144, "restart averaging (F)"="restart 3", "frequency range"="frequency range 3", "error in (no error)"=w139, "averaging type"=T15."Exponential", "exp avg settings"="exp avg settings 3") -> ("filter settled"=→"filter settled 2":bool, "octave spectrum"=→"octave graph 2":T8, "total band power"=→"Total Band Power 2":dbl, "error out"=w137:errorcluster)  [unwired: 4 in, 2 out]
        n94 = call-poly <vilib>:"SVT Sound Level.vi"("scaled signal [EU]"=w144, "integration time [s]"="integration time [s]", "measurement selection"=T16 {"Leq"=TRUE, "Running Leq"=TRUE, "Exponential"=TRUE, "Peak"=FALSE}, "exponential mode"=w143, "time constant [ms]"=w142, "error in (no error)"=w139, "restart averaging (F)"=w98) -> ("exp avg sound level [dB EU]"=w100:waveform(dbl), "Leq sound level [dB EU]"=w91:waveform(dbl), "running Leq sound level [dB EU]"=w131:waveform(dbl), "unit label"=→"unit label 2":string, "error out"=w138:errorcluster)  [unwired: 3 in, 1 out]
        "Leq sound level [dB EU] 2" <- w91
        "Exp Avg 2" <- w100
        "Running Leq sound level [dB EU] 3" <- w131
        n95 = Divide(x=w91, y=10.0) -> (x/y=w89:waveform(dbl))
        n96 = Power Of 10(x=w89) -> (10^x=w87:waveform(dbl))
        n97 = Power Of 10(x=w88) -> (10^x=w86:waveform(dbl))
        n98 = Merge Errors(w137, w138) -> (w136:errorcluster)
        n99 = Add(1:w86, 2:w87) -> (0:w84:waveform(dbl))  [unwired: 1 in, 1 out]
        n100 = Build Array(w91, w100, w131) -> (→"History 2":waveform(dbl)[])
        n101 = Unbundle By Name(w136) -> ("status"=w133:bool)
        n102 = Divide(x=w84, y=2.0) -> (x/y=w83:waveform(dbl))
        n103 = Or(x=w133, y="quit 3") -> ()  [unwired: 1 out]
        n104 = Logarithm Base 10(1:w83) -> (0:w82:waveform(dbl))
        n105 = Multiply(x=w82, y=10.0) -> (x*y=→"Leq sound level [dB EU] 4":waveform(dbl))
        n106 = call <vilib>:"Simple Error Handler.vi"("type of dialog (OK msg:1)"=w130) -> ()  [unwired: 4 in, 5 out]
        "iterations" <- w99
      }
      "error 2" <- w76
      n107 = call <vilib>:"DAQmx Stop Task.vi"("task/channels in"=w77) -> ("error out"=w78:errorcluster)  [unwired: 13 in, 1 out]
      n108 = call <vilib>:"Simple Error Handler.vi"("type of dialog (OK msg:1)"=w79, "error in (no error)"=w78) -> ()  [unwired: 3 in, 5 out]
    }
    frame #2 {
      n109 = call <vilib>:"Sound Output Clear.vi"("task ID"=w402) -> ()  [unwired: 10 in, 1 out]
    }
  }
